vi "SRV_Sensors Config GUI.vi"(11 "Sensors Config File Path in":path) -> (0 "error out":errorcluster, 1 "Cancelled?":bool, 3 "Sensors Config Filepath":path)   [LabVIEW 2014]
doc: "A Producer-Consumer two-loop state machine template. This template uses the LPD Command Queues to drive its execution.\n\nThere are several advantages such as:\n- convenient error state control\n- the ability to pass data between states/loops/VIs via a variant\n- command history which is extremely valuable in troubleshooting when an error occurs\n\n\nAuthor: Mike Schultz\n\nLogicPD, Inc\nwww.logicpd.com"
uses:
  SRV_Sensor Config Cluster.ctl
  SRV_Sensor Analog-Digital.ctl
  SRV_Sensor Sampling Mode.ctl
  SRV_Sensor View Config Cluster.ctl
  SRV_Sensors Names.ctl
  SRV_Sensor PicoC Shared Var Type.ctl
  SRV_Sensor Number of Bytes.ctl
  SRV_Sensor Integer Word Type.ctl
  SRV_Sensor Config Control refs.ctl
  Support/SRV_Command-Data Queue Data Type.ctl
panel:
  in  "Scrollbar":u32(c297)
  in  "Sensors Config GUI":T9={"Sensor Config Index 0"={"Name"="Button xx", "A/D"=enum."Analog", "I2C Address"=0, "Register"=0, "Channel"=0, "Digital Mask"=0, "Units"="", "Sampling Mode"=enum."Polled", "Sample Period (ms)"=1000, "Formula"="", "Sensor View Config"={"Sensor Name"=enum."Gauge 01", "Minimum"=0.0, "Maximum"=10.0}, "Active"=FALSE, "PicoC Shared Var Type"=enum."Integer", "Index"=0, "Stream Multiple?"=FALSE, "Index End"=255, "Bytes"=enum."1 Byte", "Source Sensor Name"="", "Repeat Start"=FALSE, "Integer Word Type"=enum."Unsigned", "Byte Swap"=FALSE}, "Sensor Config Index 1"={"Name"="Button xx", "A/D"=enum."Analog", "I2C Address"=0, "Register"=0, "Channel"=0, "Digital Mask"=0, "Units"="", "Sampling Mode"=enum."Polled", "Sample Period (ms)"=1000, "Formula"="", "Sensor View Config"={"Sensor Name"=enum."Gauge 01", "Minimum"=0.0, "Maximum"=10.0}, "Active"=FALSE, "PicoC Shared Var Type"=enum."Integer", "Index"=0, "Stream Multiple?"=FALSE, "Index End"=255, "Bytes"=enum."1 Byte", "Source Sensor Name"="", "Repeat Start"=FALSE, "Integer Word Type"=enum."Unsigned", "Byte Swap"=FALSE}, "Sensor Config Index 2"={"Name"="Button xx", "A/D"=enum."Analog", "I2C Address"=0, "Register"=0, "Channel"=0, "Digital Mask"=0, "Units"="", "Sampling Mode"=enum."Polled", "Sample Period (ms)"=1000, "Formula"="", "Sensor View Config"={"Sensor Name"=enum."Gauge 01", "Minimum"=0.0, "Maximum"=10.0}, "Active"=FALSE, "PicoC Shared Var Type"=enum."Integer", "Index"=0, "Stream Multiple?"=FALSE, "Index End"=255, "Bytes"=enum."1 Byte", "Source Sensor Name"="", "Repeat Start"=FALSE, "Integer Word Type"=enum."Unsigned", "Byte Swap"=FALSE}} {"Sensor Config Index 2"."Register" format="%.0x"; "Sensor Config Index 2"."I2C Address" format="%.0x"; "Sensor Config Index 2"."Sample Period (ms)" min=10 max=60000 step=1; "Sensor Config Index 2"."Digital Mask" format="%.0x"; "Sensor Config Index 2"."Channel" format="%.0x"; "Sensor Config Index 1"."Register" format="%.0x"; "Sensor Config Index 1"."I2C Address" format="%.0x"; "Sensor Config Index 1"."Sample Period (ms)" min=10 max=60000 step=1; "Sensor Config Index 1"."Digital Mask" format="%.0x"; "Sensor Config Index 1"."Channel" format="%.0x"; "Sensor Config Index 0"."Register" format="%.0x"; "Sensor Config Index 0"."I2C Address" format="%.0x"; "Sensor Config Index 0"."Sample Period (ms)" min=10 max=60000 step=1; "Sensor Config Index 0"."Digital Mask" format="%.0x"; "Sensor Config Index 0"."Channel" format="%.0x"}
  in  "Cancel Button":bool
  in  "OK Button":bool
  in  "About":bool
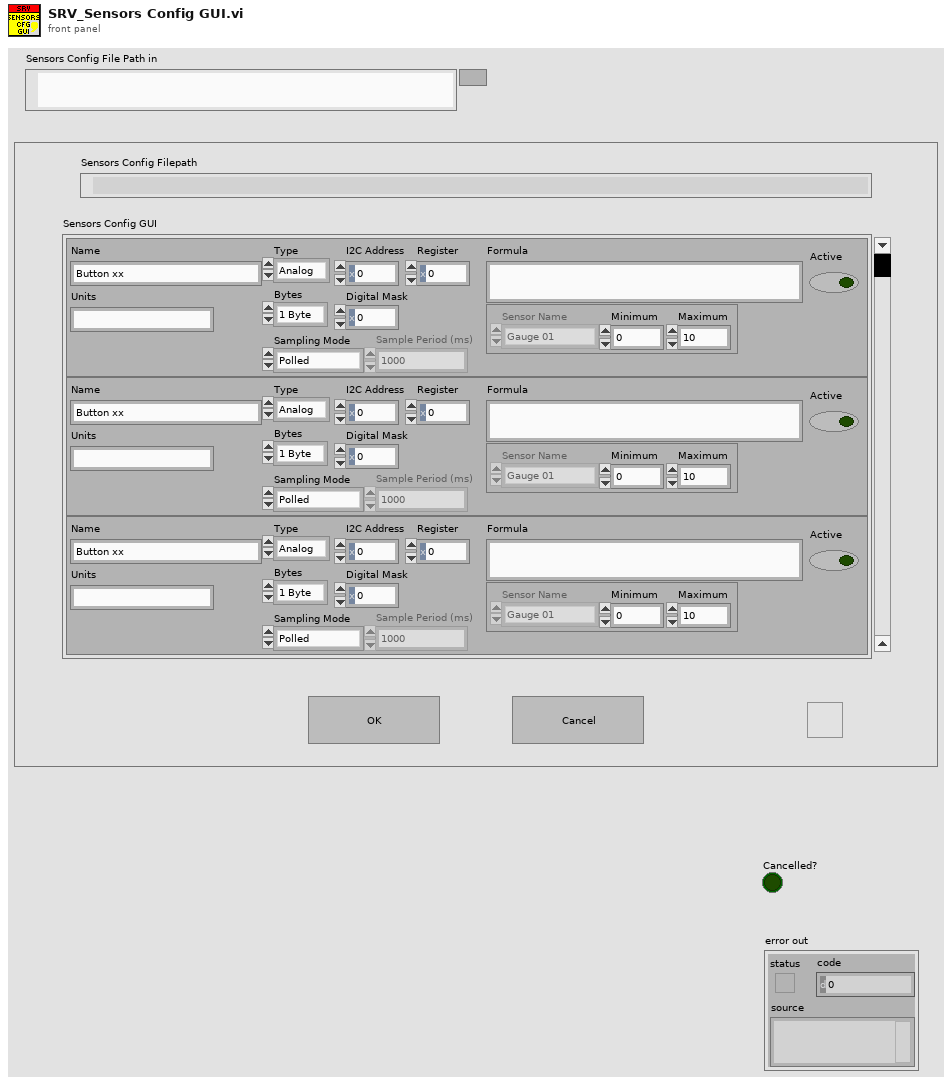
[diagram p1: front panel]
types:
  T1 = typedef "SRV_Sensor Config Cluster.ctl" = cluster{"Name":string, "A/D":T2, "I2C Address":u8, "Register":u8, "Channel":u8, "Digital Mask":u16, "Units":string, "Sampling Mode":T3, "Sample Period (ms)":u32, "Formula":string, "Sensor View Config":T4, "Active":bool, "PicoC Shared Var Type":T6, "Index":u8, "Stream Multiple?":bool, "Index End":u8, "Bytes":T7, "Source Sensor Name":string, "Repeat Start":bool, "Integer Word Type":T8, "Byte Swap":bool}
  T2 = typedef "SRV_Sensor Analog-Digital.ctl" = enum16{"Digital", "Analog", "PicoC Shared", "Calculated"}
  T3 = typedef "SRV_Sensor Sampling Mode.ctl" = enum16{"Polled", "Streaming"}
  T4 = typedef "SRV_Sensor View Config Cluster.ctl" = cluster{"Sensor Name":T5, "Minimum":dbl, "Maximum":dbl}
  T5 = typedef "SRV_Sensors Names.ctl" = enum16{"Gauge 01", "Gauge 02", "Gauge 03", "Gauge 04", "Meter 01", "Meter 02", "Meter 03", "Meter 04", "Numeric 01", "Numeric 02", "Numeric 03", "Numeric 04", "Numeric 05", "Numeric 06", "Numeric 07", "Numeric 08", "Boolean 01", "Boolean 02", "Boolean 03", "Boolean 04", "Boolean 05", "Boolean 06", "Boolean 07", "Boolean 08", "Boolean 09", "Boolean 10", "Boolean 11", "Boolean 12", "Boolean 13", "Boolean 14", "Boolean 15", "Boolean 16", "Boolean 17", "Boolean 18", "Boolean 19", "Boolean 20", "Boolean 21", "Boolean 22", "Boolean 23", "Boolean 24", "Boolean 25", "Boolean 26", "Boolean 27", "Boolean 28", "Boolean 29", "Boolean 30", "Boolean 31", "Boolean 32"}
  T6 = typedef "SRV_Sensor PicoC Shared Var Type.ctl" = enum16{"String", "Integer", "Float"}
  T7 = typedef "SRV_Sensor Number of Bytes.ctl" = enum16{"1 Byte", "2 Bytes"}
  T8 = typedef "SRV_Sensor Integer Word Type.ctl" = enum32{"Unsigned", "Signed"}
  T9 = cluster{"Sensor Config Index 0":T1, "Sensor Config Index 1":T1, "Sensor Config Index 2":T1}
  T10 = typedef "SRV_Command-Data Queue Data Type.ctl" = cluster{"Command":string, "Data":variant}
  T11 = typedef "SRV_Sensor Config Control refs.ctl" = cluster{"I2C Address refs":refnum<vi>[], "Register refs":refnum<vi>[], "Channel refs":refnum<vi>[], "Digital Mask refs":refnum<vi>[], "PicoC Shared Var Type refs":refnum<vi>[], "Index refs":refnum<vi>[], "Stream Multiple refs":refnum<vi>[], "Index End refs":refnum<vi>[], "Sample Period refs":refnum<vi>[], "Bytes refs":refnum<vi>[], "Sensor Name refs":refnum<vi>[], "Minimum refs":refnum<vi>[], "Maximum refs":refnum<vi>[], "Source Sensor Name refs":refnum<vi>[], "Sampling Mode refs":refnum<vi>[], "Repeat Start refs":refnum<vi>[], "Integer Word Type refs":refnum<vi>[], "Byte Swap refs":refnum<vi>[]}
  T12 = cluster{"user event":refnum<user-event>, "Sensor Config Filepath":path, "All Sensors Config":T1[], "Scrollbar Value":i32, "Number Display Rows":i32, "Cancelled?":bool, "Sensor Config Control refs":T11}
  T13 = enum8{"Enabled", "Disabled", "Disabled and Grayed Out"}
  T14 = cluster{"Sensor Index 0":T1, "Sensor Index 1":T1, "Sensor Index 2":T1}
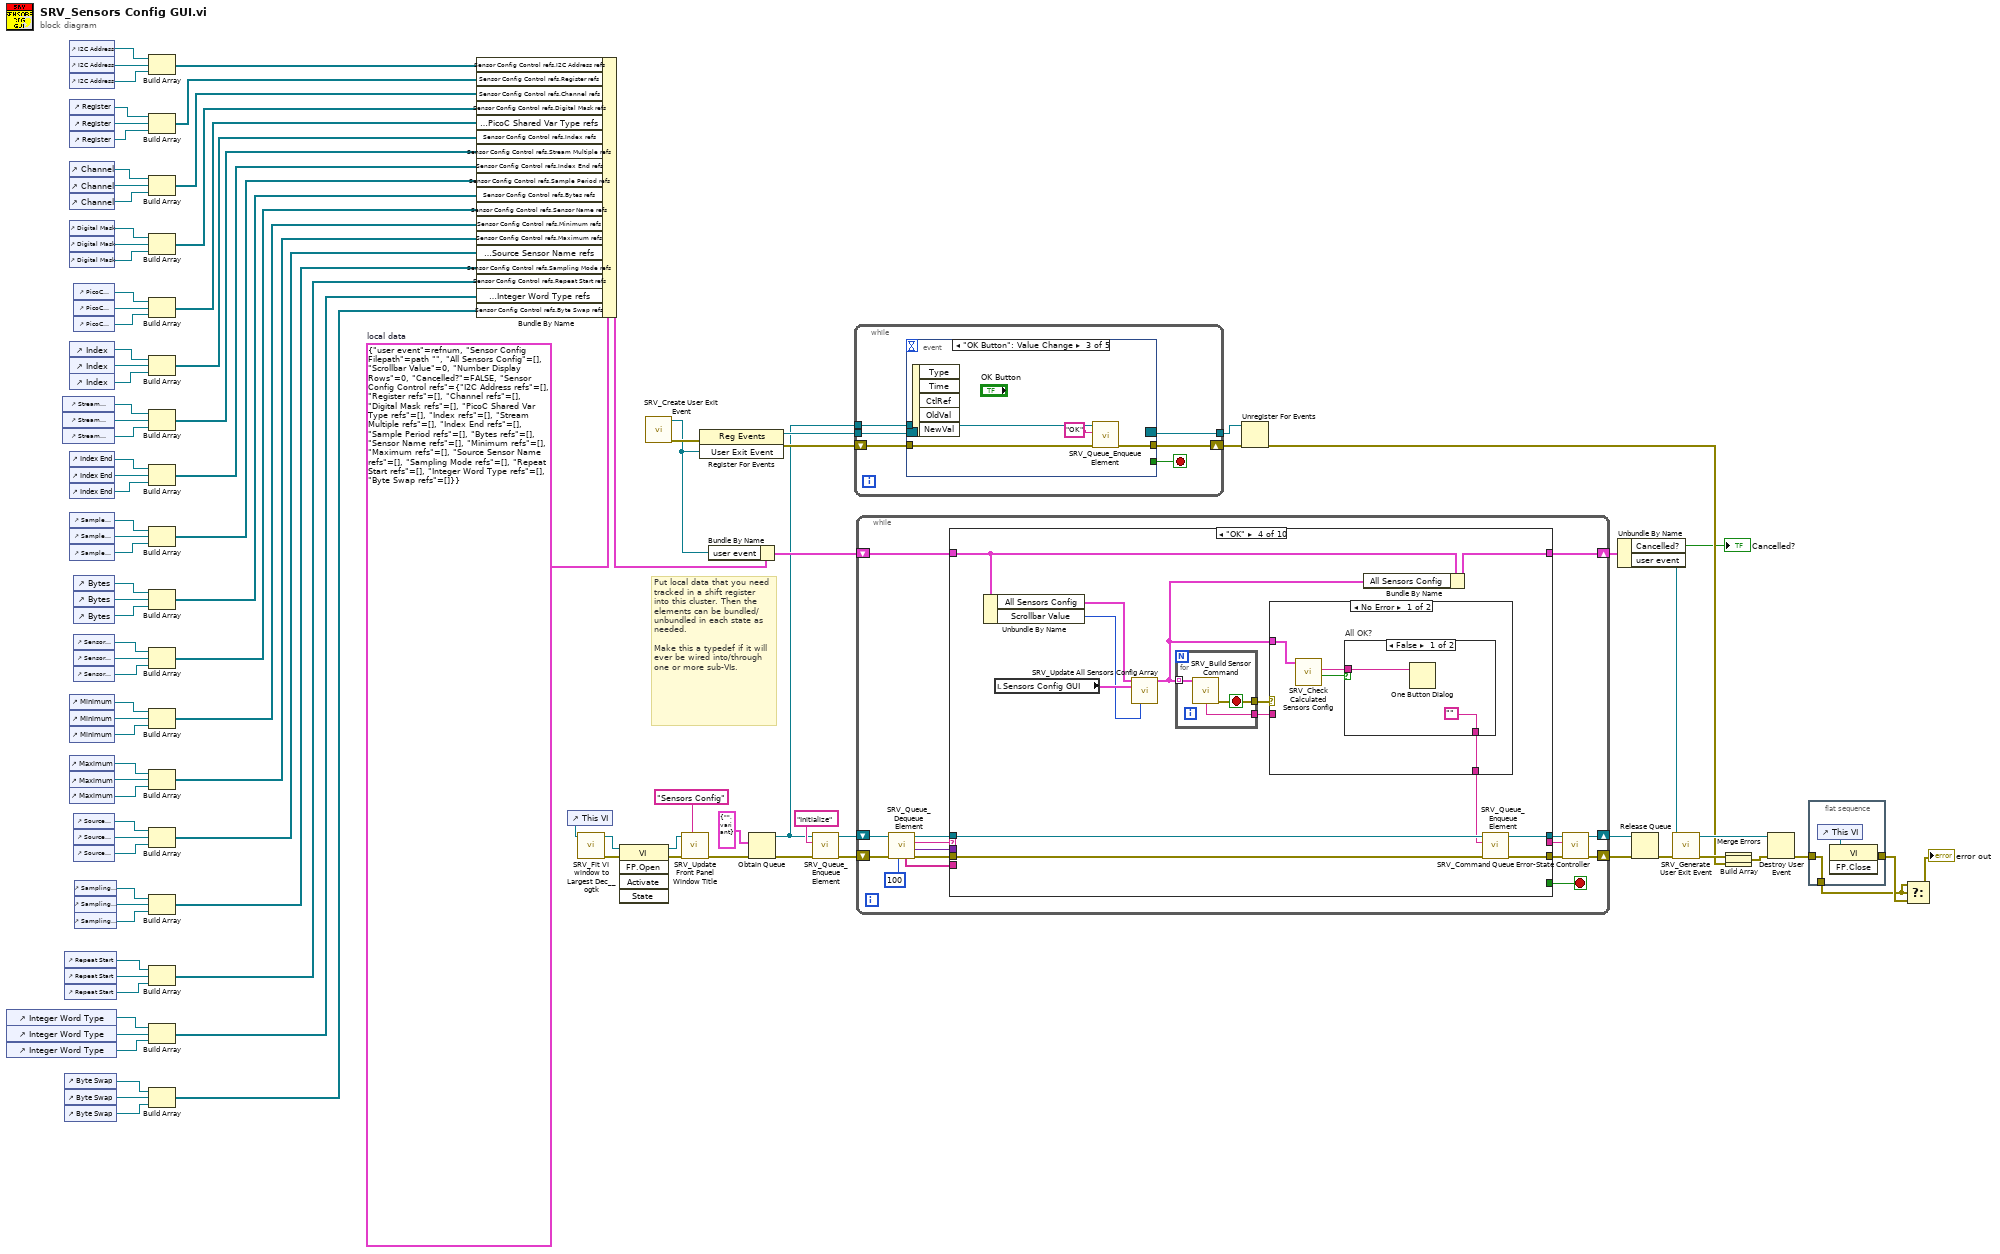
[diagram p0: block diagram]
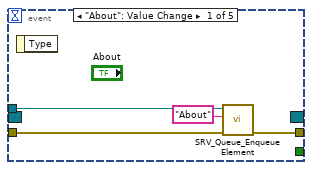
[diagram p2: hidden frame]
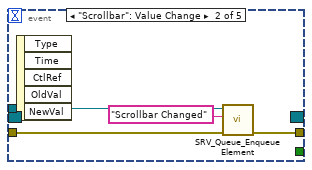
[diagram p3: hidden frame]
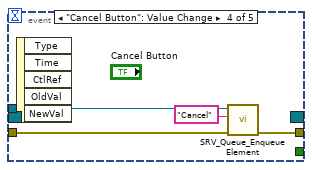
[diagram p4: hidden frame]
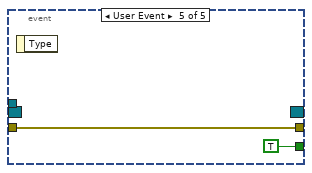
[diagram p5: hidden frame]
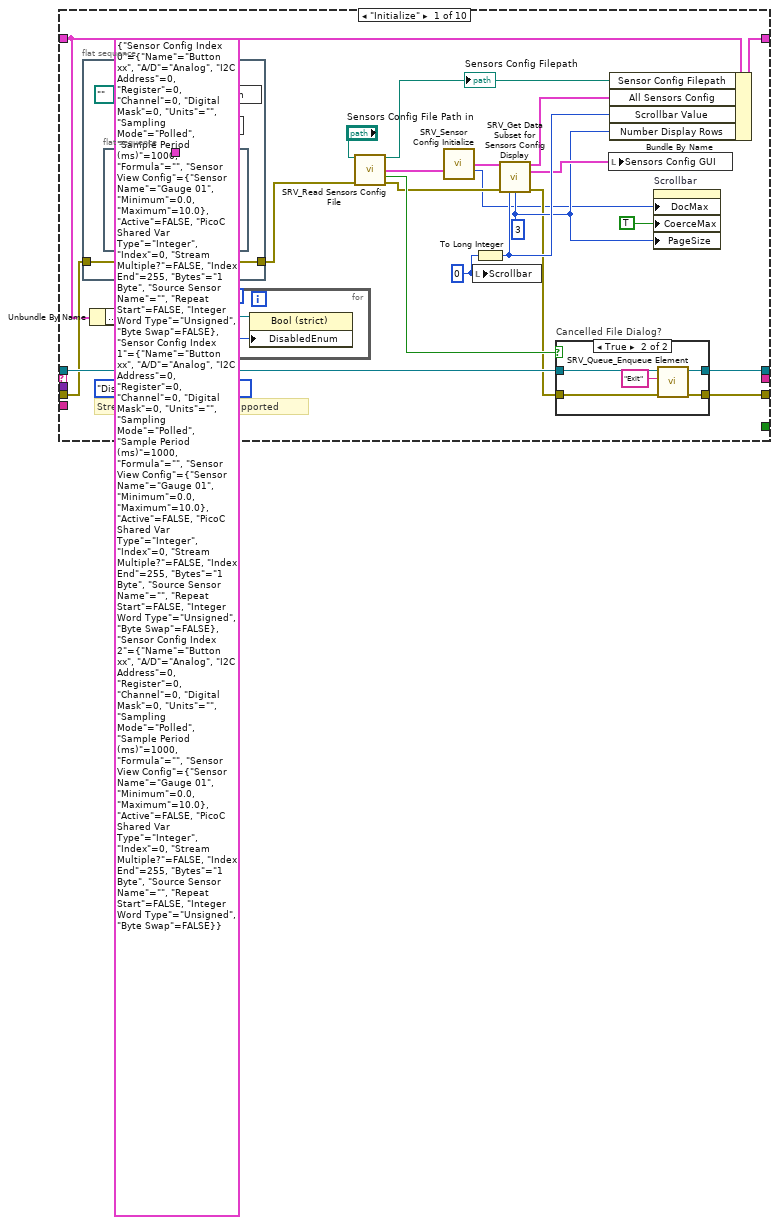
[diagram p6: hidden frame]
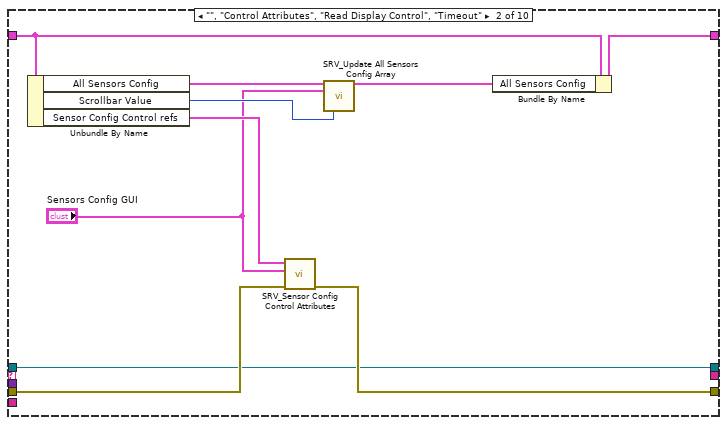
[diagram p8: hidden frame]
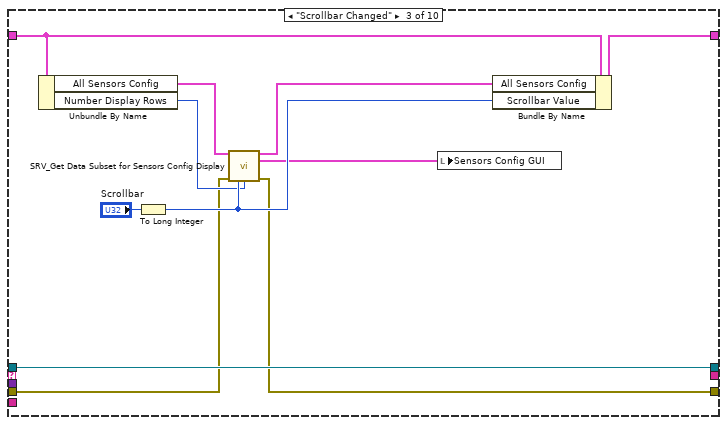
[diagram p9: hidden frame]
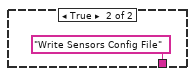
[diagram p10: hidden frame]
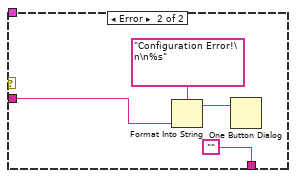
[diagram p11: hidden frame]
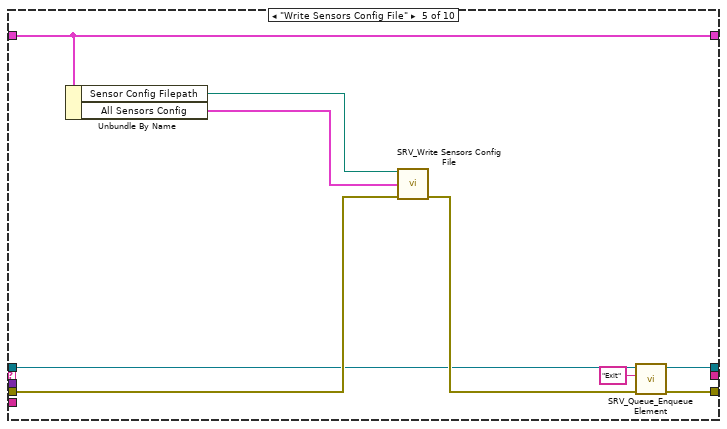
[diagram p12: hidden frame]
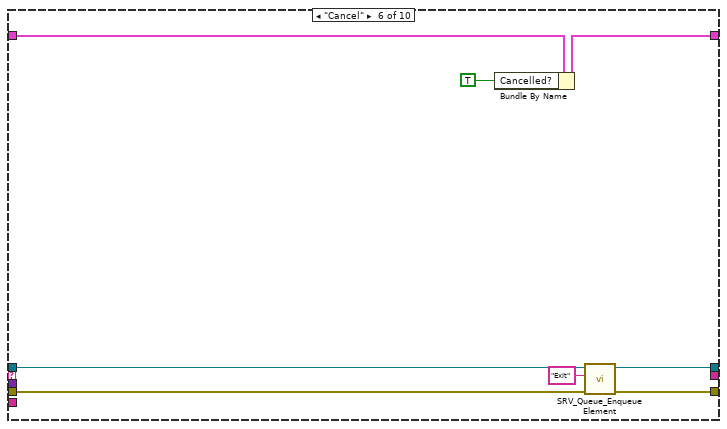
[diagram p13: hidden frame]
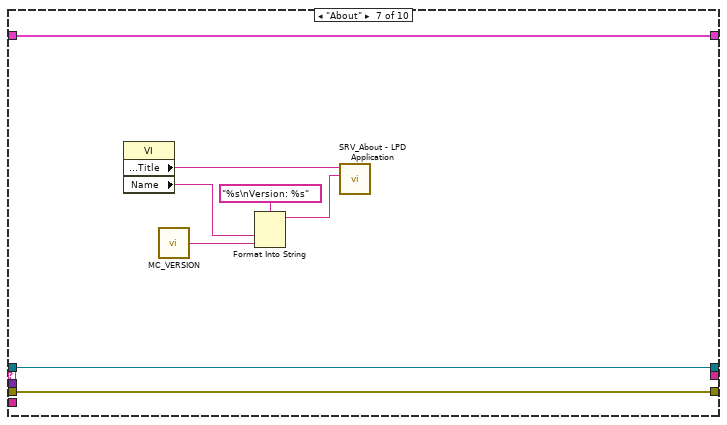
[diagram p14: hidden frame]
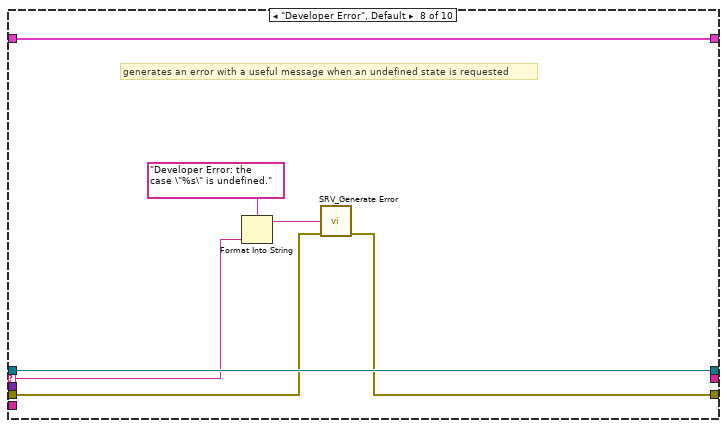
[diagram p15: hidden frame]
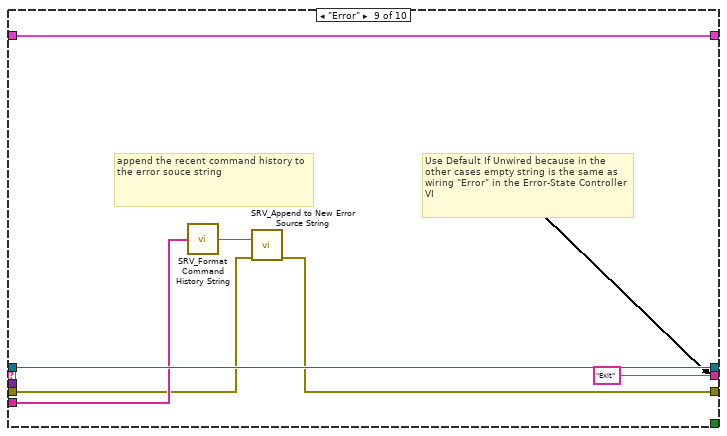
[diagram p16: hidden frame]
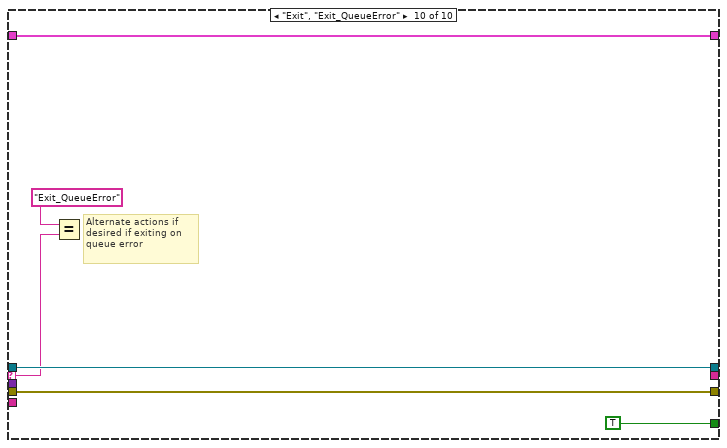
[diagram p17: hidden frame]
diagram:
  w43 = T12 {"user event"=refnum, "Sensor Config Filepath"=path "", "All Sensors Config"=[], "Scrollbar Value"=0, "Number Display Rows"=0, "Cancelled?"=FALSE, "Sensor Config Control refs"={"I2C Address refs"=[], "Register refs"=[], "Channel refs"=[], "Digital Mask refs"=[], "PicoC Shared Var Type refs"=[], "Index refs"=[], "Stream Multiple refs"=[], "Index End refs"=[], "Sample Period refs"=[], "Bytes refs"=[], "Sensor Name refs"=[], "Minimum refs"=[], "Maximum refs"=[], "Source Sensor Name refs"=[], "Sampling Mode refs"=[], "Repeat Start refs"=[], "Integer Word Type refs"=[], "Byte Swap refs"=[]}}  # local data
  # "Put local data that you need tracked in a shift register into this cluster. Then the elements can be bundled/unbundled in each state as needed.\n\nMake this a typedef if it will ever be wired into/through one or more sub-VIs."
  n1 = control-ref of="Integer Word Type"() -> (w10:refnum<vi>)
  n2 = control-ref of="Integer Word Type"() -> (w11:refnum<vi>)
  n3 = control-ref of="Integer Word Type"() -> (w9:refnum<vi>)
  n4 = control-ref of="Stream Multiple?"() -> (w73:refnum<vi>)
  n5 = control-ref of="Stream Multiple?"() -> (w74:refnum<vi>)
  n6 = control-ref of="Stream Multiple?"() -> (w72:refnum<vi>)
  n7 = control-ref of="Repeat Start"() -> (w8:refnum<vi>)
  n8 = control-ref of="Repeat Start"() -> (w12:refnum<vi>)
  n9 = control-ref of="Repeat Start"() -> (w7:refnum<vi>)
  n10 = control-ref of="Byte Swap"() -> (w3:refnum<vi>)
  n11 = control-ref of="Byte Swap"() -> (w4:refnum<vi>)
  n12 = control-ref of="Byte Swap"() -> (w2:refnum<vi>)
  n13 = control-ref of="I2C Address"() -> (w67:refnum<vi>)
  n14 = control-ref of="I2C Address"() -> (w68:refnum<vi>)
  n15 = control-ref of="I2C Address"() -> (w66:refnum<vi>)
  n16 = control-ref of="Register"() -> (w61:refnum<vi>)
  n17 = control-ref of="Register"() -> (w62:refnum<vi>)
  n18 = control-ref of="Register"() -> (w60:refnum<vi>)
  n19 = control-ref of="Channel"() -> (w58:refnum<vi>)
  n20 = control-ref of="Channel"() -> (w59:refnum<vi>)
  n21 = control-ref of="Channel"() -> (w57:refnum<vi>)
  n22 = control-ref of="Digital Mask"() -> (w55:refnum<vi>)
  n23 = control-ref of="Digital Mask"() -> (w56:refnum<vi>)
  n24 = control-ref of="Digital Mask"() -> (w54:refnum<vi>)
  n25 = control-ref of="Index"() -> (w70:refnum<vi>)
  n26 = control-ref of="Index"() -> (w71:refnum<vi>)
  n27 = control-ref of="Index"() -> (w69:refnum<vi>)
  n28 = control-ref of="Index End"() -> (w64:refnum<vi>)
  n29 = control-ref of="Index End"() -> (w65:refnum<vi>)
  n30 = control-ref of="Index End"() -> (w63:refnum<vi>)
  n31 = control-ref of="Sample Period (ms)"() -> (w40:refnum<vi>)
  n32 = control-ref of="Sample Period (ms)"() -> (w41:refnum<vi>)
  n33 = control-ref of="Sample Period (ms)"() -> (w39:refnum<vi>)
  n34 = control-ref of="Minimum"() -> (w28:refnum<vi>)
  n35 = control-ref of="Minimum"() -> (w29:refnum<vi>)
  n36 = control-ref of="Minimum"() -> (w27:refnum<vi>)
  n37 = control-ref of="Maximum"() -> (w25:refnum<vi>)
  n38 = control-ref of="Maximum"() -> (w26:refnum<vi>)
  n39 = control-ref of="Maximum"() -> (w24:refnum<vi>)
  n40 = control-ref of="PicoC Shared Var Type"() -> (w52:refnum<vi>)
  n41 = control-ref of="PicoC Shared Var Type"() -> (w53:refnum<vi>)
  n42 = control-ref of="PicoC Shared Var Type"() -> (w51:refnum<vi>)
  n43 = control-ref of="Bytes"() -> (w36:refnum<vi>)
  n44 = control-ref of="Bytes"() -> (w37:refnum<vi>)
  n45 = control-ref of="Bytes"() -> (w35:refnum<vi>)
  n46 = control-ref of="Sensor Name"() -> (w31:refnum<vi>)
  n47 = control-ref of="Sensor Name"() -> (w32:refnum<vi>)
  n48 = control-ref of="Sensor Name"() -> (w30:refnum<vi>)
  n49 = control-ref of="Source Sensor Name"() -> (w19:refnum<vi>)
  n50 = control-ref of="Source Sensor Name"() -> (w20:refnum<vi>)
  n51 = control-ref of="Source Sensor Name"() -> (w18:refnum<vi>)
  n52 = control-ref of="Sampling Mode"() -> (w16:refnum<vi>)
  n53 = control-ref of="Sampling Mode"() -> (w14:refnum<vi>)
  n54 = control-ref of="Sampling Mode"() -> (w15:refnum<vi>)
  n55 = Build Array(w67, w68, w66) -> (w50:refnum<vi>[])
  n56 = Build Array(w61, w62, w60) -> (w49:refnum<vi>[])
  n57 = Build Array(w58, w59, w57) -> (w48:refnum<vi>[])
  n58 = Build Array(w55, w56, w54) -> (w33:refnum<vi>[])
  n59 = Build Array(w52, w53, w51) -> (w47:refnum<vi>[])
  n60 = Build Array(w70, w71, w69) -> (w46:refnum<vi>[])
  n61 = Build Array(w73, w74, w72) -> (w45:refnum<vi>[])
  n62 = Build Array(w64, w65, w63) -> (w44:refnum<vi>[])
  n63 = Build Array(w40, w41, w39) -> (w38:refnum<vi>[])
  n64 = Build Array(w36, w37, w35) -> (w34:refnum<vi>[])
  n65 = Build Array(w31, w32, w30) -> (w23:refnum<vi>[])
  n66 = Build Array(w28, w29, w27) -> (w22:refnum<vi>[])
  n67 = Build Array(w25, w26, w24) -> (w21:refnum<vi>[])
  n68 = Build Array(w19, w20, w18) -> (w17:refnum<vi>[])
  n69 = Build Array(w16, w14, w15) -> (w13:refnum<vi>[])
  n70 = Build Array(w8, w12, w7) -> (w6:refnum<vi>[])
  n71 = Build Array(w10, w11, w9) -> (w5:refnum<vi>[])
  n72 = Build Array(w3, w4, w2) -> (w1:refnum<vi>[])
  n73 = Bundle By Name(cluster=w43, "Sensor Config Control refs.I2C Address refs"=w50, "Sensor Config Control refs.Register refs"=w49, "Sensor Config Control refs.Channel refs"=w48, "Sensor Config Control refs.Digital Mask refs"=w33, "Sensor Config Control refs.PicoC Shared Var Type refs"=w47, "Sensor Config Control refs.Index refs"=w46, "Sensor Config Control refs.Stream Multiple refs"=w45, "Sensor Config Control refs.Index End refs"=w44, "Sensor Config Control refs.Sample Period refs"=w38, "Sensor Config Control refs.Bytes refs"=w34, "Sensor Config Control refs.Sensor Name refs"=w23, "Sensor Config Control refs.Minimum refs"=w22, "Sensor Config Control refs.Maximum refs"=w21, "Sensor Config Control refs.Source Sensor Name refs"=w17, "Sensor Config Control refs.Sampling Mode refs"=w13, "Sensor Config Control refs.Repeat Start refs"=w6, "Sensor Config Control refs.Integer Word Type refs"=w5, "Sensor Config Control refs.Byte Swap refs"=w1) -> (w42:T12)
  n74 = control-ref of="This VI"() -> (w79:refnum<vi>)
  n75 = call "SRV_Fit VI window to Largest Dec__ogtk.vi"("VI Ref (calling VI)"=w79) -> ("error out"=w82:errorcluster, "dup VI Ref"=w78:refnum<vi>)  [unwired: 5 in]
  n76 = invoke class="VI" method="FP.Open"(reference=w78, error in=w82) -> (reference out=w75:refnum<vi>, error out=w77:errorcluster)  [unwired: 3 in, 3 out]
  n77 = call "SRV_Create User Exit Event.vi"() -> ("error out"=w95:errorcluster, "User Exit Event"=w94:refnum<user-event>)  [unwired: 10 in]
  n78 = call "SRV_Update Front Panel Window Title.vi"("Window Title Override String"="Sensors Config", "error in (no error)"=w77, "VI ref"=w75) -> ("error out"=w76:errorcluster)  [unwired: 7 in, 1 out]
  n79 = register-events(error in=w95, w94) -> (reference out=w109:refnum<event-registration>, error out=w108:errorcluster)  [unwired: 1 in]
  n80 = Bundle By Name(cluster=w42, "user event"=w94) -> (w103:T12)
  n81 = Obtain Queue(element data type=T10 {"Command"="", "Data"=variant} ("Queue Data Type"), error in (no error)=w76) -> (queue out=w90:refnum<queue>, error out=w91:errorcluster)  [unwired: 3 in, 1 out]
  n82 = call "SRV_Queue_Enqueue Element.vi"("error in (no error)"=w91, "Command"="Initialize", "Command-Data Queue"=w90) -> ("error out"=w87:errorcluster, "Command-Data Queue out"=w89:refnum<queue>)  [unwired: 6 in, 1 out]
  n83 = while {
    shift-right: [w114] -> w106
    shift-left: w108 -> [w115]
    tunnel: w90 -> [w113]
    tunnel: w109 -> [w112]
    tunnel: [w111] -> w107
    stop <- w110 stop-if-true
    n84 = event shown="[2] \"OK Button\": Value Change" {
      selector: w112 -> [_ _ _ _ _]
      dyn-events: [_ _ _ _ _] -> w111
      timeout: _ -> [_ _ _ _ _]
      tunnel: w115 -> [w119 w123 w125 w129 w133]
      tunnel: [w118 w122 w126 w130 w133] -> w114
      tunnel: w113 -> [w116 w120 w124 w128 _]
      tunnel: [_ _ _ _ TRUE] -> w110
      event "About": Value Change {
        n85 = event-data() -> ()  [unwired: 1 in, 1 out]
        n86 = call "SRV_Queue_Enqueue Element.vi"("error in (no error)"=w119, "Command"="About", "Command-Data Queue"=w116) -> ("error out"=w118:errorcluster)  [unwired: 6 in, 2 out]
      }
      event "Scrollbar": Value Change {
        n87 = event-data() -> ()  [unwired: 1 in, 5 out]
        n88 = call "SRV_Queue_Enqueue Element.vi"("error in (no error)"=w123, "Command"="Scrollbar Changed", "Command-Data Queue"=w120) -> ("error out"=w122:errorcluster)  [unwired: 6 in, 2 out]
      }
      event "OK Button": Value Change {
        n89 = event-data() -> ()  [unwired: 1 in, 5 out]
        n90 = call "SRV_Queue_Enqueue Element.vi"("error in (no error)"=w125, "Command"="OK", "Command-Data Queue"=w124) -> ("error out"=w126:errorcluster)  [unwired: 6 in, 2 out]
      }
      event "Cancel Button": Value Change {
        n91 = event-data() -> ()  [unwired: 1 in, 5 out]
        n92 = call "SRV_Queue_Enqueue Element.vi"("error in (no error)"=w129, "Command"="Cancel", "Command-Data Queue"=w128) -> ("error out"=w130:errorcluster)  [unwired: 6 in, 2 out]
      }
      event User Event {
        n93 = event-data() -> ()  [unwired: 1 in, 1 out]
      }
    }
  }
  n94 = while {
    shift-right: [w143] -> w105
    shift-left: w87 -> [w149]
    shift-right: [w141] -> w104
    shift-left: w89 -> [w147]
    shift-right: [w135] -> w102
    shift-left: w103 -> [w136]
    stop <- w137 stop-if-true
    n95 = call "SRV_Queue_Dequeue Element.vi"("timeout in ms (-1)"=100, "error in (no error)"=w149, "Command-Data Queue"=w147) -> ("error out"=w148:errorcluster, "Data"=w140:variant, "Command"=w145:string, "Command-Data Queue out"=w146:refnum<queue>, "Command History"=w139:string[])  [unwired: 3 in, 1 out]
    n96 = case shown="\"OK\"" w145 {
      selector: w145 -> [_ _ _ _ _ _ _ w263 _ w275]
      tunnel: w148 -> [w165 w193 w198 w211 w241 w249 w257 w261 w267 w277]
      tunnel: [w170 w187 w197 w219 w238 w248 w257 w260 w268 w277] -> w144
      tunnel: w146 -> [w171 w186 w206 w218 w237 w250 w258 w265 w272 w278]
      tunnel: [w169 w186 w206 w217 w236 w247 w258 w265 w272 w278] -> w142
      tunnel: w140 -> [_ _ _ _ _ _ _ _ _ _]
      tunnel: w139 -> [_ _ _ _ _ _ _ _ w271 _]
      tunnel: [_ _ _ _ _ _ _ _ "Exit" ("Error Command") _] -> w138
      tunnel: [_ _ _ _ _ _ _ _ _ TRUE] -> w137
      tunnel: w136 -> [w150 w194 w204 w213 w234 w245 w252 w262 w269 w273]
      tunnel: [w168 w195 w205 w212 w234 w244 w252 w262 w269 w273] -> w135
      frame "Initialize" {
        w159 = 3 ("Number Display Rows")
        w163 = u32 0 ("Scrollbar")
        # "Streaming multiple not yet supported"
        n97 = flat-sequence {
          tunnel: [w176] -> w166
          tunnel: w165 -> [w176]
          frame #0 {
            n98 = flat-sequence {
              tunnel: [T9 {"Sensor Config Index 0"={"Name"="Button xx", "A/D"=enum."Analog", "I2C Address"=0, "Register"=0, "Channel"=0, "Digital Mask"=0, "Units"="", "Sampling Mode"=enum."Polled", "Sample Period (ms)"=1000, "Formula"="", "Sensor View Config"={"Sensor Name"=enum."Gauge 01", "Minimum"=0.0, "Maximum"=10.0}, "Active"=FALSE, "PicoC Shared Var Type"=enum."Integer", "Index"=0, "Stream Multiple?"=FALSE, "Index End"=255, "Bytes"=enum."1 Byte", "Source Sensor Name"="", "Repeat Start"=FALSE, "Integer Word Type"=enum."Unsigned", "Byte Swap"=FALSE}, "Sensor Config Index 1"={"Name"="Button xx", "A/D"=enum."Analog", "I2C Address"=0, "Register"=0, "Channel"=0, "Digital Mask"=0, "Units"="", "Sampling Mode"=enum."Polled", "Sample Period (ms)"=1000, "Formula"="", "Sensor View Config"={"Sensor Name"=enum."Gauge 01", "Minimum"=0.0, "Maximum"=10.0}, "Active"=FALSE, "PicoC Shared Var Type"=enum."Integer", "Index"=0, "Stream Multiple?"=FALSE, "Index End"=255, "Bytes"=enum."1 Byte", "Source Sensor Name"="", "Repeat Start"=FALSE, "Integer Word Type"=enum."Unsigned", "Byte Swap"=FALSE}, "Sensor Config Index 2"={"Name"="Button xx", "A/D"=enum."Analog", "I2C Address"=0, "Register"=0, "Channel"=0, "Digital Mask"=0, "Units"="", "Sampling Mode"=enum."Polled", "Sample Period (ms)"=1000, "Formula"="", "Sensor View Config"={"Sensor Name"=enum."Gauge 01", "Minimum"=0.0, "Maximum"=10.0}, "Active"=FALSE, "PicoC Shared Var Type"=enum."Integer", "Index"=0, "Stream Multiple?"=FALSE, "Index End"=255, "Bytes"=enum."1 Byte", "Source Sensor Name"="", "Repeat Start"=FALSE, "Integer Word Type"=enum."Unsigned", "Byte Swap"=FALSE}} ("Sensors Config GUI")] -> w175
              frame #0 {
              }
            }
            n99 = local write "Sensors Config Filepath"(path "" ("Sensor Config Filepath")) -> ()
            n100 = local write "Sensors Config GUI"(w175) -> ()
          }
        }
        n101 = Unbundle By Name(w150) -> ("Sensor Config Control refs.Stream Multiple refs"=w152:refnum<vi>[])
        n102 = for {
          tunnel: w152 -> [w174] mode=indexing
          tunnel: T13."Disabled and Grayed Out" ("Disabled") -> [w173]
          n103 = property class="Bool (strict)"(reference=w174, "DisabledEnum"=w173) -> ()  [unwired: 1 in, 2 out]
        }
        n104 = call "SRV_Read Sensors Config File.vi"("Sensors Config File Path"="Sensors Config File Path in", "error in (no error)"=w166) -> ("Sensors Config File Path out"=w167:path, "Sensors Config"=w155:T1[], "Cancelled?"=w172:bool, "error out"=w157:errorcluster)  [unwired: 10 in]
        "Sensors Config Filepath" <- w167
        n105 = call "SRV_Sensor Config Initialize.vi"("Sensors Config"=w155) -> ("Sensors Config out"=w154:T1[], "Number of Sensors"=w153:i32)  [unwired: 13 in]
        n106 = local write "Scrollbar"(w163) -> ()
        n107 = To Long Integer(number=w163) -> (32bit integer=w162:i32)
        n108 = call "SRV_Get Data Subset for Sensors Config Display.vi"("All Sensors Config"=w154, "error in (no error)"=w157, "Row Start Index"=w162, "Number of Rows to Display (3)"=w159) -> ("All Sensors Config dup"=w164:T1[], "Sensors Config GUI"=w161:T14, "error out"=w156:errorcluster)  [unwired: 9 in]
        n109 = case "Cancelled File Dialog?" shown="True" w172 {
          tunnel: w156 -> [w179 w184]
          tunnel: w171 -> [w180 w185]
          tunnel: [w179 w183] -> w170
          tunnel: [w180 w182] -> w169
          frame False {
          }
          frame True {
            n110 = call "SRV_Queue_Enqueue Element.vi"("error in (no error)"=w184, "Command"="Exit", "Command-Data Queue"=w185) -> ("error out"=w183:errorcluster, "Command-Data Queue out"=w182:refnum<queue>)  [unwired: 6 in, 1 out]
          }
        }
        n111 = local write "Sensors Config GUI"(w161) -> ()
        n112 = Bundle By Name(cluster=w150, "Sensor Config Filepath"=w167, "All Sensors Config"=w164, "Scrollbar Value"=w162, "Number Display Rows"=w159) -> (w168:T12)
        n113 = property on="Scrollbar" class="Scroll (strict)"("DocMax"=w153, "CoerceMax"=TRUE ("Coerce Maximum Value"), "PageSize"=w159) -> ()  [unwired: 2 in, 2 out]
      }
      frame "", "Control Attributes", "Read Display Control", "Timeout" {
        n114 = Unbundle By Name(w194) -> ("All Sensors Config"=w191:T1[], "Scrollbar Value"=w189:i32, "Sensor Config Control refs"=w192:T11)
        n115 = call "SRV_Sensor Config Control Attributes.vi"("error in (no error)"=w193, "Sensors Config GUI"="Sensors Config GUI", "Sensor Config Control refs"=w192) -> ("error out"=w187:errorcluster)  [unwired: 8 in]
        n116 = call "SRV_Update All Sensors Config Array.vi"("All Sensors Config"=w191, "Sensors Config GUI"="Sensors Config GUI", "Row Start Index"=w189) -> ("All Sensors Config out"=w190:T1[])  [unwired: 12 in]
        n117 = Bundle By Name(cluster=w194, "All Sensors Config"=w190) -> (w195:T12)
      }
      frame "Scrollbar Changed" {
        n118 = Unbundle By Name(w204) -> ("All Sensors Config"=w196:T1[], "Number Display Rows"=w199:i32)
        n119 = To Long Integer(number="Scrollbar") -> (32bit integer=w202:i32)
        n120 = call "SRV_Get Data Subset for Sensors Config Display.vi"("All Sensors Config"=w196, "error in (no error)"=w198, "Row Start Index"=w202, "Number of Rows to Display (3)"=w199) -> ("All Sensors Config dup"=w201:T1[], "Sensors Config GUI"=w200:T14, "error out"=w197:errorcluster)  [unwired: 9 in]
        n121 = local write "Sensors Config GUI"(w200) -> ()
        n122 = Bundle By Name(cluster=w204, "All Sensors Config"=w201, "Scrollbar Value"=w202) -> (w205:T12)
      }
      frame "OK" {
        n123 = Unbundle By Name(w213) -> ("All Sensors Config"=w214:T1[], "Scrollbar Value"=w215:i32)
        n124 = local read "Sensors Config GUI"() -> (w216:T9)
        n125 = call "SRV_Update All Sensors Config Array.vi"("All Sensors Config"=w214, "Sensors Config GUI"=w216, "Row Start Index"=w215) -> ("All Sensors Config out"=w207:T1[])  [unwired: 12 in]
        n126 = for {
          tunnel: w207 -> [w233] mode=indexing
          tunnel: [w232] -> w210
          tunnel: [w231] -> w208
          stop <- w232 stop-if-true
          n127 = call "SRV_Build Sensor Command.vi"("Sensor Config"=w233) -> ("Error Message"=w231:string, "error out"=w232:errorcluster)  [unwired: 9 in, 4 out]
        }
        n128 = case shown="No Error" w210 {
          tunnel: [w221 ""] -> w209
          tunnel: w208 -> [_ w229]
          tunnel: w207 -> [w223 _]
          frame No Error {
            n129 = call "SRV_Check Calculated Sensors Config.vi"("All Sensors Config"=w223) -> ("All OK?"=w222:bool, "Error Message String"=w220:string)  [unwired: 9 in]
            n130 = case "All OK?" shown="False" w222 {
              tunnel: ["" "Write Sensors Config File" ("Command")] -> w221
              tunnel: w220 -> [w224 _]
              frame False {
                n131 = One Button Dialog(message=w224) -> ()  [unwired: 1 in, 1 out]
              }
              frame True {
              }
            }
          }
          frame Error {
            n132 = Format Into String(format string="Configuration Error!\n\n%s", w229) -> (resulting string=w227:string)  [unwired: 2 in, 1 out]
            n133 = One Button Dialog(message=w227) -> ()  [unwired: 1 in, 1 out]
          }
        }
        n134 = Bundle By Name(cluster=w213, "All Sensors Config"=w207) -> (w212:T12)
        n135 = call "SRV_Queue_Enqueue Element.vi"("error in (no error)"=w211, "Command"=w209, "Command-Data Queue"=w218) -> ("error out"=w219:errorcluster, "Command-Data Queue out"=w217:refnum<queue>)  [unwired: 6 in, 1 out]
      }
      frame "Write Sensors Config File" {
        n136 = Unbundle By Name(w234) -> ("Sensor Config Filepath"=w242:path, "All Sensors Config"=w235:T1[])
        n137 = call "SRV_Write Sensors Config File.vi"("Sensors Config File Path"=w242, "Sensors Config"=w235, "error in (no error)"=w241) -> ("error out"=w239:errorcluster)  [unwired: 12 in]
        n138 = call "SRV_Queue_Enqueue Element.vi"("error in (no error)"=w239, "Command"="Exit", "Command-Data Queue"=w237) -> ("error out"=w238:errorcluster, "Command-Data Queue out"=w236:refnum<queue>)  [unwired: 6 in, 1 out]
      }
      frame "Cancel" {
        n139 = Bundle By Name(cluster=w245, "Cancelled?"=TRUE) -> (w244:T12)
        n140 = call "SRV_Queue_Enqueue Element.vi"("error in (no error)"=w249, "Command"="Exit", "Command-Data Queue"=w250) -> ("error out"=w248:errorcluster, "Command-Data Queue out"=w247:refnum<queue>)  [unwired: 6 in, 1 out]
      }
      frame "About" {
        n141 = property class="VI"() -> ("Front Panel.Title"=w256:string, "Name"=w253:string)  [unwired: 2 in, 2 out]
        n142 = call "MC_VERSION.vi"() -> ("MC Version"=w251:string)
        n143 = Format Into String(format string="%s\nVersion: %s", w253, w251) -> (resulting string=w254:string)  [unwired: 2 in, 1 out]
        n144 = call "SRV_About - LPD Application.vi"("Version Info"=w254, "Application Name"=w256) -> ()  [unwired: 10 in]
      }
      frame "Developer Error", Default {
        # "generates an error with a useful message when an undefined state is requested"
        n145 = Format Into String(format string="Developer Error: the case \"%s\" is undefined.", w263) -> (resulting string=w259:string)  [unwired: 2 in, 1 out]
        n146 = call "SRV_Generate Error.vi"("Message"=w259, "error in (no error)"=w261) -> ("error out"=w260:errorcluster)  [unwired: 13 in]
      }
      frame "Error" {
        # "Use Default If Unwired because in the other cases empty string is the same as wiring \"Error\" in the Error-State Controller VI"
        # "append the recent command history to the error souce string"
        n147 = call "SRV_Format Command History String.vi"("Command History"=w271) -> ("Command History String"=w266:string)  [unwired: 14 in]
        n148 = call "SRV_Append to New Error Source String.vi"("Message String to append"=w266, "Error In (no error)"=w267) -> ("error out"=w268:errorcluster)  [unwired: 13 in]
      }
      frame "Exit", "Exit_QueueError" {
        # "Alternate actions if desired if exiting on queue error"
        n149 = Equal?(x="Exit_QueueError", y=w275) -> ()  [unwired: 1 out]
      }
    }
    n150 = call "SRV_Command Queue Error-State Controller.vi"("error in (no error)"=w144, "Error Command"=w138, "Command-Data Queue"=w142) -> ("error out"=w143:errorcluster, "Command-Data Queue out"=w141:refnum<queue>)  [unwired: 7 in]
  }
  n151 = Unregister For Events(event registration refnum=w107, error in=w106) -> (error out=w97:errorcluster)
  n152 = Unbundle By Name(w102) -> ("Cancelled?"=→"Cancelled?":bool, "user event"=w101:refnum<user-event>)
  n153 = Release Queue(queue=w104, error in (no error)=w105) -> (error out=w100:errorcluster)  [unwired: 1 in, 2 out]
  n154 = call "SRV_Generate User Exit Event.vi"("error in (no error)"=w100, "User Exit Event"=w101) -> ("error out"=w98:errorcluster, "User Exit Event out"=w99:refnum<user-event>)  [unwired: 8 in]
  n155 = Build Array(w98, w97) -> (w93:errorcluster[])
  n156 = Merge Errors(w93) -> (w96:errorcluster)
  n157 = Destroy User Event(user event=w99, error in=w96) -> (error out=w84:errorcluster)
  n158 = flat-sequence {
    tunnel: [w280] -> w86
    tunnel: w84 -> [w279]
    tunnel: [w279] -> w83
    frame #0 {
      n159 = control-ref of="This VI"() -> (w281:refnum<vi>)
      n160 = invoke class="VI" method="FP.Close"(reference=w281) -> (error out=w280:errorcluster)  [unwired: 2 in, 2 out]
    }
  }
  n161 = Select(t=w83, s=w83, f=w86) -> (s? t:f=→"error out":errorcluster)
